vi "Init Panel Array.vi"(8 "error in (no error)":errorcluster, 11 "GVIWebProcessorApp in":refnum<class "GVIWebProcessorApp.lvclass">) -> (0 "error out":errorcluster, 3 "GVIWebProcessorApp out":refnum<class "GVIWebProcessorApp.lvclass">)   [LabVIEW 2020, in "PicoG-Processor.lvlib" / "GVIWebProcessorApp.lvclass"]
uses:
  GVIWebProcessorApp.lvclass
  GVIWebProcessorApp.lvclass/GVIWebProcessorApp.ctl
  <vilib>/IlluminatedG/IG OOPanel/OOPanel/ArrayManager/ArrayManager.lvclass
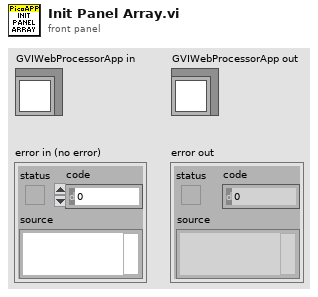
[diagram p1: front panel]
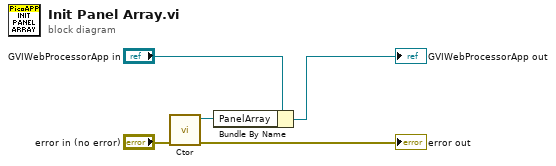
[diagram p0: block diagram]
diagram:
  n1 = call <vilib>:"Ctor.vi"("error in (no error)"="error in (no error)") -> ("error out"=→"error out":errorcluster, "PanelArray"=w3:refnum<class "ArrayManager.lvclass">)  [unwired: 9 in]
  n2 = Bundle By Name(cluster="GVIWebProcessorApp in", "PanelArray"=w3) -> (→"GVIWebProcessorApp out":refnum<class "GVIWebProcessorApp.lvclass">)
